vi "Get TCP Connection.vi"(8 "error in (no error)":errorcluster, 11 "TCP Client in":refnum<class "TCP Client.lvclass">) -> (0 "error out":errorcluster, 2 "TCP Connection":refnum<k5>, 3 "TCP Client out":refnum<class "TCP Client.lvclass">)   [LabVIEW 2024, in "Stream-TCP.lvlib" / "TCP Client.lvclass"]
uses:
  TCP Client.lvclass
  TCP Client.lvclass/TCP Client.ctl
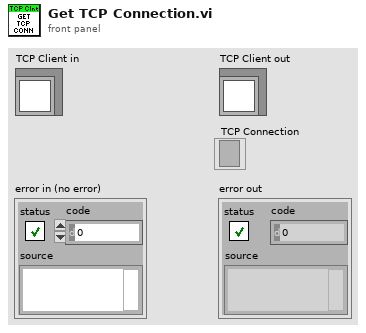
[diagram p1: front panel]
types:
  T1 = typedef "Stream-TCP.lvlib/TCP Client.lvclass/Ref Data.ctl" = cluster{"TCP Connection":refnum<k5>, "TCP Stream":refnum<class "TCP Stream.lvclass">, "Connection Loop":refnum<vi>, "Timeout ms":i32, "Server Connection":bool, "Open":bool}
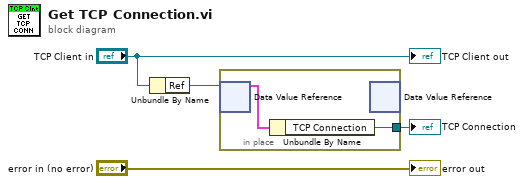
[diagram p0: block diagram]
diagram:
  n1 = Unbundle By Name("TCP Client in") -> ("Ref"=w3:refnum<data-value>)
  n2 = in-place {
    in-place-border: [w5] -> w1
    n3 = in-place-dvr #1(w3) -> (w6:T1)  [unwired: 1 out]
    n4 = Unbundle By Name(w6) -> ("TCP Connection"=w5:refnum<k5>)
    n5 = in-place-dvr #1() -> ()  [unwired: 1 in, 2 out]
  }
  "TCP Connection" <- w1
  "error out" <- "error in (no error)"
  "TCP Client out" <- "TCP Client in"
